vi "Read Multiple Analog Channels.vi"(8 "error in":errorcluster, 9 "Channel Selection":T2(array[ring]), 10 "Voltage Data":bool=TRUE, 11 "VISA resource name":refnum<visa-resource-name>) -> (0 "error out":errorcluster, 2 "Channel Data":dbl[](array[numeric]), 3 "VISA resource name":refnum<visa-resource-name>)   [LabVIEW 2020, in "BDAQ-6104.lvlib"]
uses:
  <instrlib>/BDAQ-6104/BDAQ-6104.lvlib
panel:
  out "Channel Number":T1(ring)
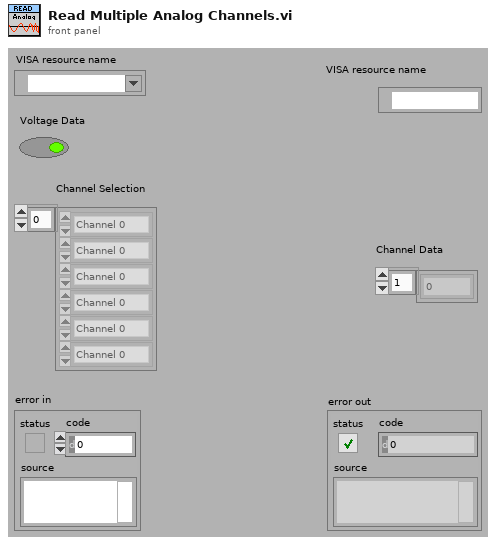
[diagram p1: front panel]
types:
  T1 = enum16{"Channel 0", "Channel 1", "Channel 2", "Channel 3", "Channel 4", "Channel 5"}
  T2 = enum16{"Channel 0", "Channel 1", "Channel 2", "Channel 3", "Channel 4", "Channel 5"}[]
  T3 = cluster{"AIO-0":dbl, "AIO-1":dbl, "AIO-2":dbl, "AIO-3":dbl, "AIO-4":dbl, "AIO-5":dbl}
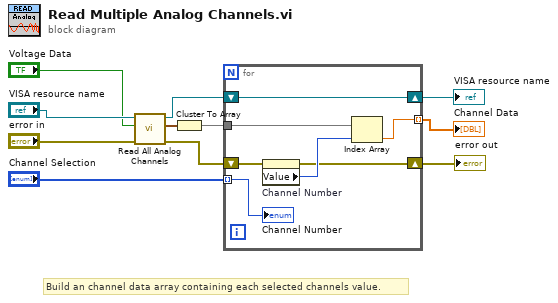
[diagram p0: block diagram]
diagram:
  # "Build an channel data array containing each selected channels value."
  n1 = call <instrlib>:"Read All Analog Channels.vi"("error in"="error in", "Voltage Data"="Voltage Data", "VISA resource name"="VISA resource name") -> ("error out"=w2:errorcluster, "Analog output cluster"=w11:T3, "VISA resource name out"=w4:refnum<visa-resource-name>)  [unwired: 5 in]
  n2 = Cluster To Array(cluster=w11) -> (array=w9:dbl[])
  n3 = for {
    tunnel: "Channel Selection" -> [w15] mode=indexing
    tunnel: w9 -> [w18]
    tunnel: [w17] -> w8 mode=indexing
    shift-right: [w16] -> w3
    shift-left: w4 -> [w16]
    shift-right: [w12] -> w1
    shift-left: w2 -> [w13]
    n4 = property on="Channel Number" class="Enum (strict)"(error in=w13) -> (error out=w12:errorcluster, "Value"=w14:T1)  [unwired: 1 in, 1 out]
    n5 = Index Array(array=w18, index=w14) -> (element=w17:dbl)
    "Channel Number" <- w15
  }
  "Channel Data" <- w8
  "VISA resource name" <- w3
  "error out" <- w1
